vi "Tear Down.vi"(8 "error in (no error)":errorcluster, 11 "Car Wash Console in":refnum<class "Car Wash Console.lvclass">) -> (0 "error out":errorcluster, 3 "Car Wash Console out":refnum<class "Car Wash Console.lvclass">)   [LabVIEW 2016, in "CLD Exam - Car Wash.lvlib" / "Car Wash Console.lvclass"]
uses:
  Car Wash Console.lvclass
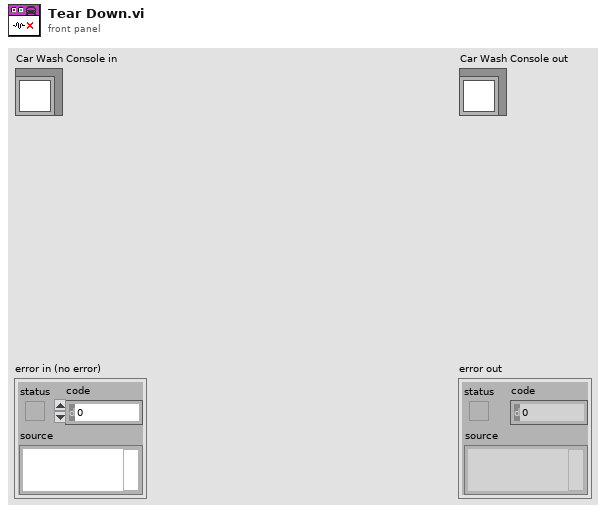
[diagram p1: front panel]
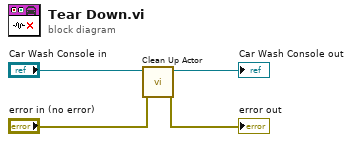
[diagram p0: block diagram]
diagram:
  n1 = call-dynamic "Clean Up Actor.vi"("error in (no error)"="error in (no error)", "Car Wash Console in"="Car Wash Console in") -> ("error out"=→"error out":errorcluster, "Car Wash Console out"=→"Car Wash Console out":refnum<class "Car Wash Console.lvclass">)  [unwired: 8 in]
